vi "Actor Core.vi"(8 "error in":errorcluster, 11 "Nested in":refnum<class "Root Actor.lvclass">) -> (0 "error out":errorcluster, 3 "Actor out":refnum<class "Actor.lvclass">)   [LabVIEW 2021, in "Root Actor.lvlib" / "Root Actor.lvclass"]
doc: "(<B>Filename</B>: Actor Framework.lvlib:Actor.lvclass:Actor Core.vi)\n\nReceives messages to the actor, reacts to them, and initiates any error handling that may shut the actor down.\n\nDescendant classes may override this VI to append parallel tasks for the actor to complete while it handles messages. Overrides use the Call Parent Method node."
uses:
  Root Actor.lvclass
  <vilib>/ActorFramework/Actor/Actor.lvclass
  <vilib>/ActorFramework/Stop Msg/Stop Msg.lvclass
  Chef States/INIT/INIT.lvclass
  Root Actor Messages/Change State To COOKING Msg/Change State To COOKING Msg.lvclass
panel:
  out "State String":string
  in  "Exit Button":bool
  in  "Start Button":bool
  # "Current State"
  # "Made by Ramazan Burak Korkmaz- 2024"
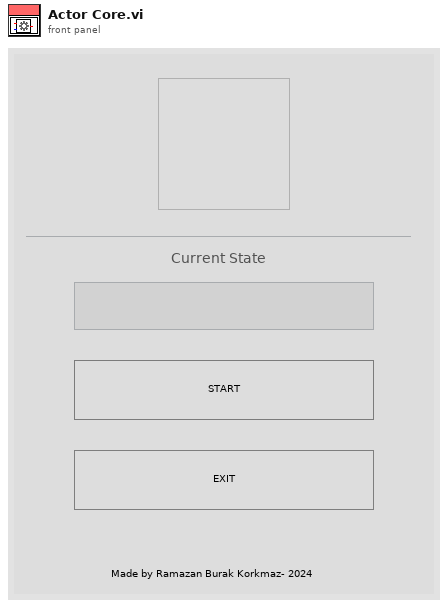
[diagram p1: front panel]
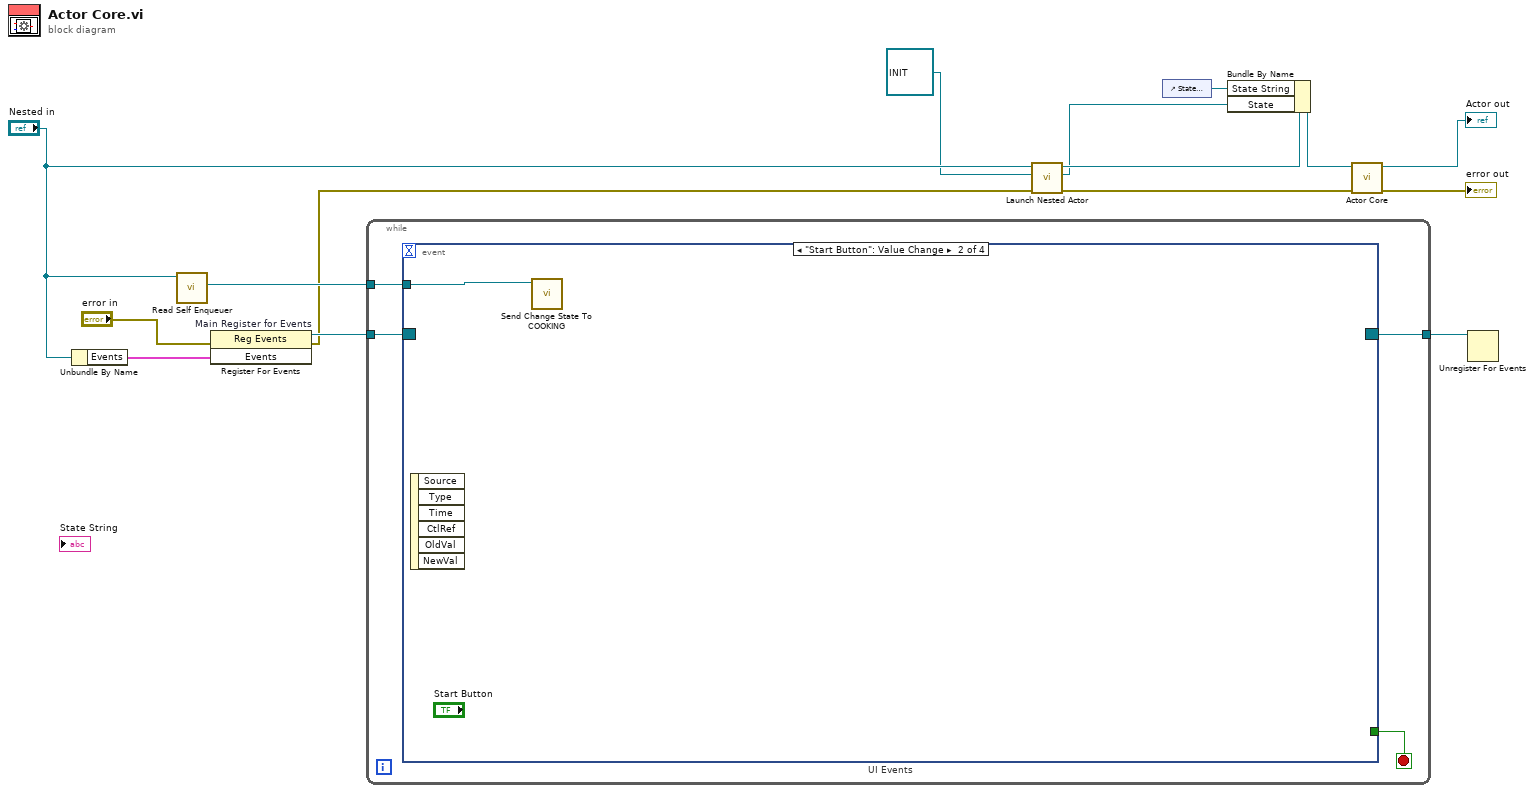
[diagram p0: block diagram]
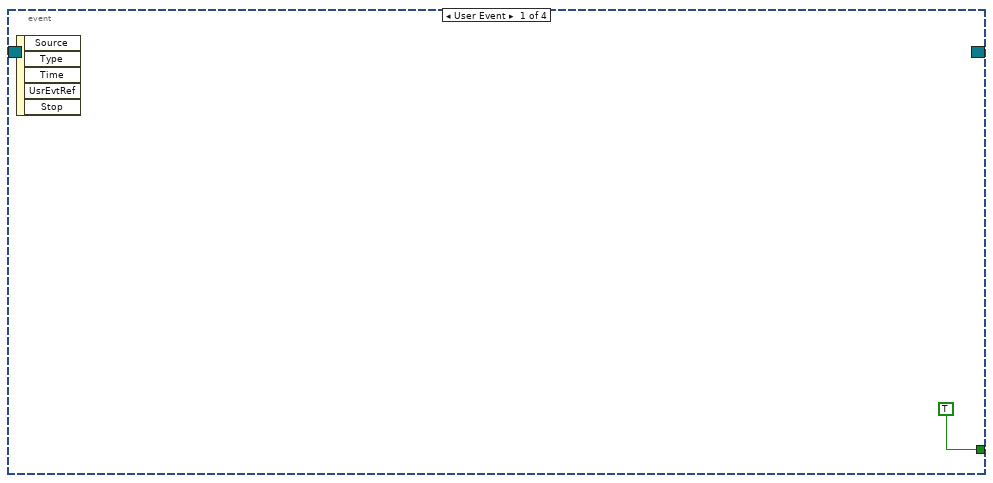
[diagram p2: hidden frame]
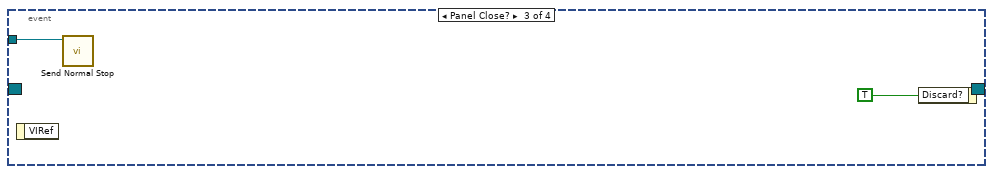
[diagram p3: hidden frame]
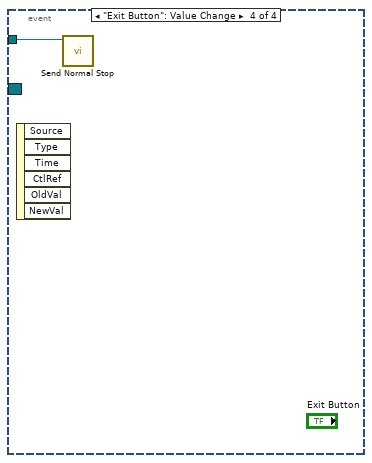
[diagram p4: hidden frame]
diagram:
  n1 = Unbundle By Name("Nested in") -> ("Events"=w12:cluster{"Stop":refnum<user-event>})
  n2 = call <vilib>:"Read Self Enqueuer.vi"("Actor"="Nested in") -> ("Self Enqueuer"=w10:refnum<class "Message Enqueuer.lvclass">)  [unwired: 10 in]
  n3 = register-events "Main Register for Events"(error in="error in", w12) -> (reference out=w13:refnum<event-registration>, error out=w8:errorcluster)  [unwired: 1 in]
  n4 = while {
    tunnel: w13 -> [w19]
    tunnel: [w17] -> w11
    tunnel: w10 -> [w16]
    stop <- w18 stop-if-true
    n5 = event "UI Events" shown="[1] \"Start Button\": Value Change" {
      selector: w19 -> [_ _ _ _]
      dyn-events: [_ _ _ _] -> w17
      timeout: _ -> [_ _ _ _]
      tunnel: [TRUE _ _ _] -> w18
      tunnel: w16 -> [_ w21 w22 w24]
      event User Event {
        n6 = event-data() -> ()  [unwired: 1 in, 5 out]
      }
      event "Start Button": Value Change {
        n7 = event-data() -> ()  [unwired: 1 in, 6 out]
        n8 = call "Send Change State To COOKING.vi"("Message Enqueuer"=w21) -> ()  [unwired: 9 in, 2 out]
      }
      event Panel Close? {
        n9 = event-data() -> ()  [unwired: 1 in, 1 out]
        n10 = call <vilib>:"Send Normal Stop.vi"("Message Enqueuer"=w22) -> ()  [unwired: 10 in, 1 out]
        n11 = event-data("Discard?"=TRUE) -> ()  [unwired: 1 in, 1 out]
      }
      event "Exit Button": Value Change {
        n12 = event-data() -> ()  [unwired: 1 in, 6 out]
        n13 = call <vilib>:"Send Normal Stop.vi"("Message Enqueuer"=w24) -> ()  [unwired: 10 in, 1 out]
      }
    }
  }
  n14 = call <vilib>:"Launch Nested Actor.vi"("error in (no error)"=w8, "Nested Actor"=refnum<class "INIT.lvclass"> refnum ("Chef States.lvlib:INIT.lvclass"), "Caller Actor in"="Nested in") -> ("error out"=w5:errorcluster, "Nested Actor's Enqueuer"=w1:refnum<class "Message Enqueuer.lvclass">, "Caller Actor out"=w6:refnum<class "Root Actor.lvclass">)  [unwired: 6 in]
  n15 = control-ref of="State String"() -> (w2:refnum<vi>)
  n16 = Bundle By Name(cluster=w6, "State String"=w2, "State"=w1) -> (w3:refnum<class "Root Actor.lvclass">)
  n17 = call-parent "Actor Core.vi"("error in"=w5, "Actor in"=w3) -> ("error out"=→"error out":errorcluster, "Actor out"=→"Actor out":refnum<class "Actor.lvclass">)  [unwired: 8 in]
  n18 = Unregister For Events(event registration refnum=w11) -> ()  [unwired: 1 in, 1 out]
